vi "KnifeEdgeExpt.vi"(7 "Rep. Rate (Hz)":dbl=1000.0 min=0.0 max=34.0, 10 "Start Position":dbl[](array[numeric]) min=0.0 max=34.0) -> (0 "SDG_Ctrl":bool, 1 "start/end points":cluster{dbl, dbl, dbl}[][](array[cluster]), 2 "Canceled":bool, 3 "Angle_Incident":dbl caption="Incident\nAngle (deg)", 4 "X/Y (T:Y)":bool=TRUE, 5 "ImageParameter":T1)   [LabVIEW 2013]
uses:
  ImagingMS/ImageConvPara_3d.ctl
  <vilib>/Native 3D Graph/xcontrol/3DPC_SurfacePlot.xctl
panel:
  in  "MainAixalStepWidth":dbl=0.01 caption="Y StepWidth"
  out "3D Graph":refnum<class "Base Datatype.lvclass">[](xcontrol)
  in  "x ? y":bool=TRUE
  in  "IncidentAngle":dbl caption="Incident\nAngle (deg)"
  in  "SDG Ctrl?":bool=TRUE
  out "Estimated Time (min)":dbl min=0.0 max=34.0
  in  "Average":i32=10 min=20 max=1000 step=20
  in  "Apply":bool
  in  "Cancel":bool
  in  "Run":bool
  out "2ndAxialSize":dbl caption="Z Size (mm)" min=0.0 max=34.0
  out "MainAxialSize":dbl caption="X Size (mm)" min=0.0 max=34.0
  in  "2ndAxialSteps":i32=20 caption="Z Steps" min=0 max=65535 step=1
  in  "MainAxialSize":dbl=0.5 caption="Y Size" min=0.0 max=34.0
  in  "2ndAxialStepWidth":dbl=0.04 caption="Z StepWidth" min=0.0 max=34.0
  # "Unit is mm always."
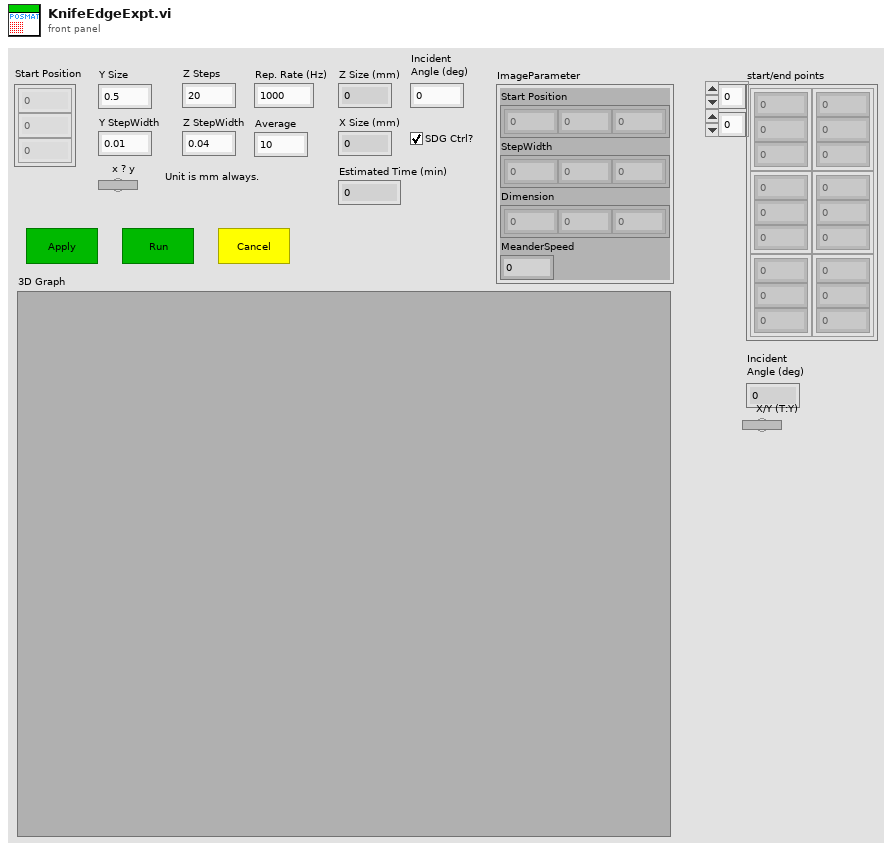
[diagram p1: front panel]
types:
  T1 = typedef "ImageConvPara_3d.ctl" = cluster{"Start Position":dbl[], "StepWidth":dbl[], "Dimension":i32[], "MeanderSpeed":dbl}
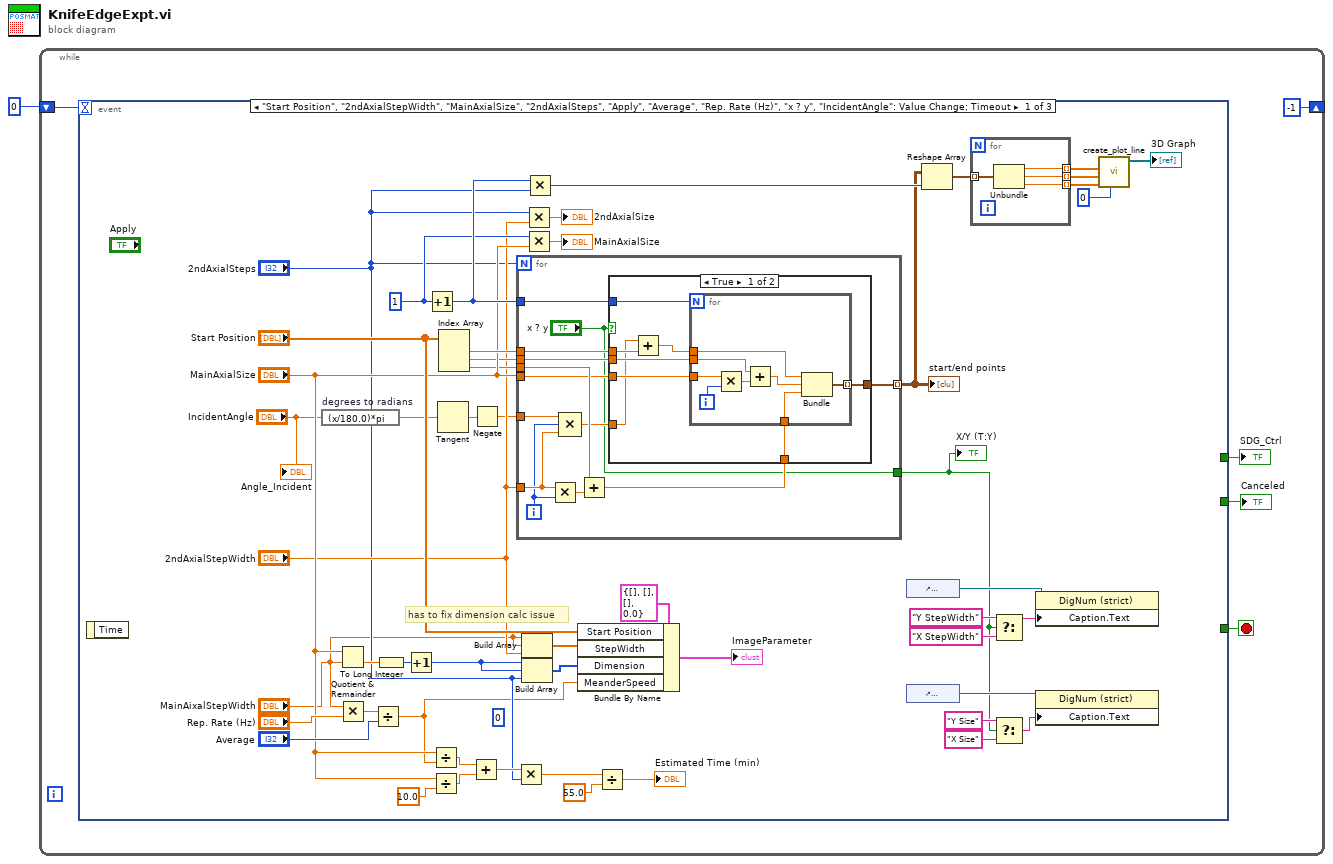
[diagram p0: block diagram]
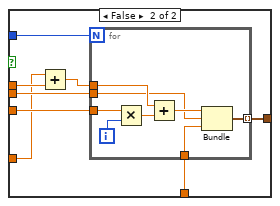
[diagram p2: hidden frame]
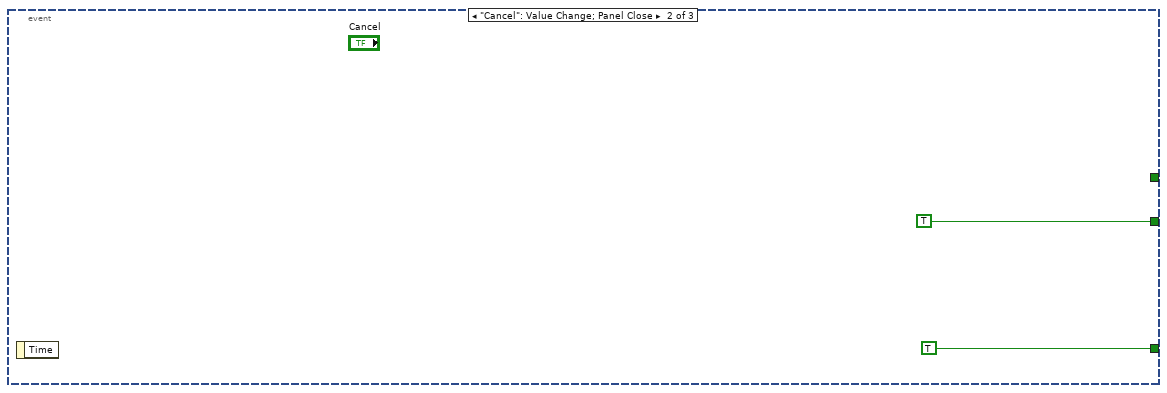
[diagram p3: hidden frame]
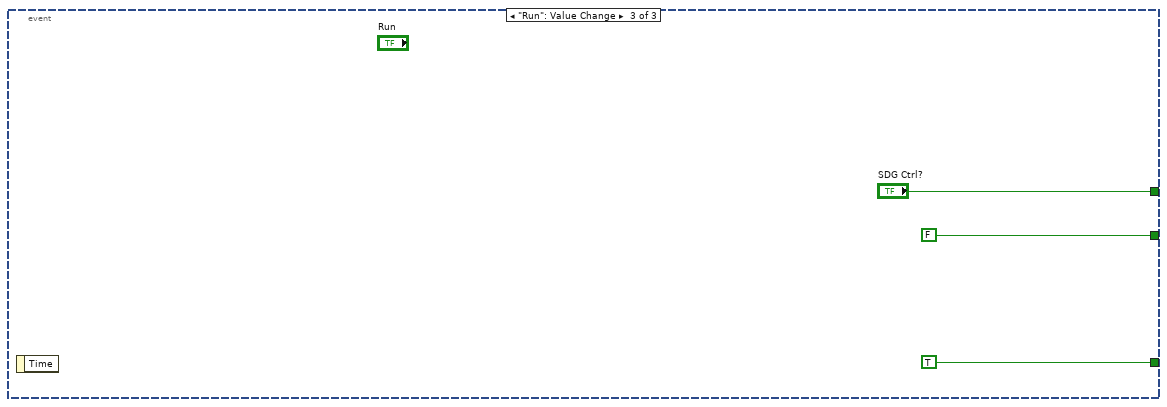
[diagram p4: hidden frame]
diagram:
  n1 = while {
    shift-right: [-1] -> _
    shift-left: 0 -> [w3]
    stop <- w6 stop-if-true
    n2 = event shown="[0] \"Start Position\", \"2ndAxialStepWidth\", \"MainAxialSize\", \"2ndAxialSteps\", \"Apply\", \"Average\", \"Rep. Rate (Hz)\", \"x ? y\", \"IncidentAngle\": Value Change;  Timeout" {
      selector: _ -> [_ _ _]
      dyn-events: _ -> [_ _ _]
      timeout: w3 -> [_ _ _]
      tunnel: [_ TRUE TRUE] -> w6
      tunnel: [_ TRUE ("Canceled") FALSE ("Canceled")] -> w5
      tunnel: [_ _ "SDG Ctrl?"] -> w4
      event "Start Position", "2ndAxialStepWidth", "MainAxialSize", "2ndAxialSteps", "Apply", "Average", "Rep. Rate (Hz)", "x ? y", "IncidentAngle": Value Change; Timeout {
        (unwired) 0 ("element")
        w52 = 1
        # "has to fix dimension calc issue"
        n3 = event-data() -> ()  [unwired: 1 in, 1 out]
        n4 = expression code="(x/180.0)*pi" "degrees to radians"("IncidentAngle") -> (w26:dbl)
        n5 = Quotient & Remainder(x="MainAxialSize", y="MainAixalStepWidth") -> (floor(x/y)=w45:dbl)  [unwired: 1 out]
        n6 = Multiply(x="MainAixalStepWidth", y="Rep. Rate (Hz)") -> (x*y=w18:dbl)
        n7 = Divide(x=w18, y="Average") -> (x/y=w29:dbl)
        n8 = To Long Integer(number=w45) -> (32bit integer=w46:i32)
        n9 = Increment(x=w46) -> (x+1=w9:i32)
        n10 = Increment(x=w52) -> (x+1=w53:i32)
        n11 = Divide(x="MainAxialSize", y=w29) -> (x/y=w41:dbl)
        n12 = Divide(x="MainAxialSize", y=10.0) -> (x/y=w40:dbl)
        n13 = Tangent(1:w26) -> (0:w28:dbl)
        n14 = Index Array(array="Start Position") -> (element #1=w57:dbl, element #2=w33:dbl, element #3=w34:dbl)  [unwired: 3 in]
        n15 = Add(x=w41, y=w40) -> (x+y=w39:dbl)
        n16 = Negate(x=w28) -> (-x=w27:dbl)
        n17 = Multiply(x=w39, y="2ndAxialSteps") -> (x*y=w38:dbl)
        n18 = for {
          N: "2ndAxialSteps" -> [_]
          tunnel: w34 -> [w70]
          tunnel: "2ndAxialStepWidth" -> [w65]
          tunnel: "MainAxialSize" -> [w69]
          tunnel: w53 -> [w72]
          tunnel: [w71] -> w32 mode=indexing
          tunnel: w27 -> [w66]
          tunnel: w57 -> [w68]
          tunnel: w33 -> [w67]
          tunnel: ["x ? y"] -> w7
          i -> [w64]
          n19 = Multiply(x=w65, y=w64) -> (x*y=w74:dbl)
          n20 = Compound Arithmetic op=MULTIPLY(w66, w64, w65) -> (w63:dbl)
          n21 = Add(x=w70, y=w74) -> (x+y=w73:dbl)
          n22 = case shown="True" "x ? y" {
            tunnel: w73 -> [w82 w98]
            tunnel: w72 -> [w81 w97]
            tunnel: [w80 w96] -> w71
            tunnel: w69 -> [w79 w95]
            tunnel: w68 -> [w77 w93]
            tunnel: w67 -> [w78 w94]
            tunnel: w63 -> [w75 w91]
            frame True {
              n23 = Add(x=w75, y=w77) -> (x+y=w76:dbl)
              n24 = for {
                N: w81 -> [_]
                tunnel: w79 -> [w88]
                tunnel: w76 -> [w83]
                tunnel: w82 -> [w86]
                tunnel: [w87] -> w80 mode=indexing
                tunnel: w78 -> [w85]
                i -> [w89]
                n25 = Multiply(x=w88, y=w89) -> (x*y=w90:dbl)
                n26 = Add(x=w85, y=w90) -> (x+y=w84:dbl)
                n27 = Bundle(w83, w84, w86) -> (w87:cluster{dbl, dbl, dbl})  [unwired: 1 in]
              }
            }
            frame False {
              n28 = Add(x=w91, y=w93) -> (x+y=w92:dbl)
              n29 = for {
                N: w97 -> [_]
                tunnel: w95 -> [w104]
                tunnel: w92 -> [w100]
                tunnel: w98 -> [w101]
                tunnel: [w103] -> w96 mode=indexing
                tunnel: w94 -> [w99]
                i -> [w105]
                n30 = Multiply(x=w104, y=w105) -> (x*y=w106:dbl)
                n31 = Add(x=w100, y=w106) -> (x+y=w102:dbl)
                n32 = Bundle(w102, "X StepWidth"=w99, w101) -> (w103:cluster{dbl, "X StepWidth":dbl, dbl})  [unwired: 1 in]
              }
            }
          }
        }
        "start/end points" <- w32
        "X/Y (T:Y)" <- w7
        n33 = Build Array("MainAixalStepWidth", "MainAixalStepWidth", "2ndAxialStepWidth") -> (w49:dbl[])
        n34 = Build Array(w9, w9, "2ndAxialSteps") -> (w48:i32[])
        n35 = Multiply(x="2ndAxialSteps", y="2ndAxialStepWidth") -> (x*y=→"2ndAxialSize":dbl)
        n36 = Multiply(x=w52, y="MainAxialSize") -> (x*y=→"MainAxialSize":dbl)
        n37 = Multiply(x=w53, y="2ndAxialSteps") -> (x*y=w54:i32)
        n38 = Bundle By Name(cluster=T1 {"Start Position"=[], "StepWidth"=[], "Dimension"=[], "MeanderSpeed"=0.0} ("ImageParameter"), "Start Position"="Start Position", "StepWidth"=w49, "Dimension"=w48, "MeanderSpeed"=w29) -> (→"ImageParameter":T1)
        n39 = Divide(x=w38, y=55.0) -> (x/y=→"Estimated Time (min)":dbl)
        n40 = control-ref of="MainAixalStepWidth"() -> (w17:refnum<vi>)
        n41 = control-ref of="MainAxialSize"() -> (w16:refnum<vi>)
        n42 = Reshape Array(w32, w54) -> (w19:cluster{dbl, "X StepWidth":dbl, dbl}[])
        n43 = for {
          tunnel: w19 -> [w61] mode=indexing
          tunnel: [w60] -> w22 mode=indexing
          tunnel: [w59] -> w23 mode=indexing
          tunnel: [w58] -> w24 mode=indexing
          n44 = Unbundle(w61) -> (w60:dbl, "X StepWidth"=w59:dbl, w58:dbl)
        }
        n45 = Select(t="Y StepWidth" ("Label.Text"), s=w7, f="X StepWidth" ("Label.Text")) -> (s? t:f=w15:string)
        n46 = Select(t="Y Size" ("Label.Text"), s=w7, f="X Size" ("Label.Text")) -> (s? t:f=w10:string)
        n47 = property class="DigNum (strict)"(reference=w17, "Caption.Text"=w15) -> ()  [unwired: 1 in, 2 out]
        n48 = property class="DigNum (strict)"(reference=w16, "Caption.Text"=w10) -> ()  [unwired: 1 in, 2 out]
        n49 = call <vilib>:"create_plot_line.vi"("plot ID"=0, "z vector"=w24, "y vector"=w23, "x vector"=w22) -> ("plots out"=→"3D Graph":refnum<class "Base Datatype.lvclass">[])  [unwired: 1 in, 6 out]
        "Angle_Incident" <- "IncidentAngle"
      }
      event "Cancel": Value Change; Panel Close {
        n50 = event-data() -> ()  [unwired: 1 in, 1 out]
      }
      event "Run": Value Change {
        n51 = event-data() -> ()  [unwired: 1 in, 1 out]
      }
    }
    "Canceled" <- w5
    "SDG_Ctrl" <- w4
  }
